vi "Disconnect and Close.vi"(0 "NI Digital in":refnum<k15>, 11 "error in (no error)":errorcluster) -> (15 "error out":errorcluster)   [LabVIEW 2018, in "Digital.lvlib"]
uses:
  Digital.lvlib
  <instrlib>/niDigital/niDigital.llb/niDigital Selected Function.ctl
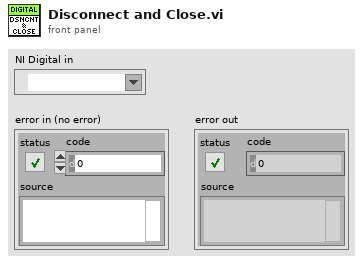
[diagram p1: front panel]
types:
  T1 = typedef "niDigital Selected Function.ctl" = i32
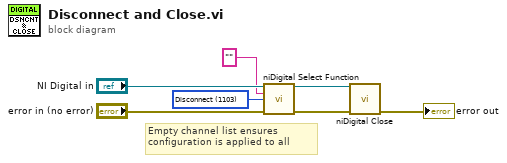
[diagram p0: block diagram]
diagram:
  w4 = T1 1103 items=["Digital"=1100, "PPMU"=1101, "Off"=1102, "Disconnect"=1103] ("function")
  # "Empty channel list ensures configuration is applied to all"
  n1 = call <instrlib>:"niDigital Select Function.vi"("instrument handle"="NI Digital in", "channel list"="", "function"=w4, "error in"="error in (no error)") -> ("instrument handle out"=w2:refnum<k15>, "error out"=w6:errorcluster)  [unwired: 10 in]
  n2 = call <instrlib>:"niDigital Close.vi"("instrument handle"=w2, "error in"=w6) -> ("error out"=→"error out":errorcluster)  [unwired: 13 in]
